vi "VA CoAP - Server - Proccess Message - SET Value TO JSON.vi"(8 "error in (no error)":errorcluster, 9 "New Value":string, 10 "Item name":string[](array[string]), 11 "JSON Value in":refnum<class "JSON Value.lvclass">) -> (0 "error out":errorcluster, 3 "JSON Value out":refnum<class "JSON Value.lvclass">)   [LabVIEW 2020]
uses:
  <vilib>/addons/JSON API/JSON Value/JSON Value.lvclass
  <vilib>/addons/JSON API/JSON Scalar/JSON Scalar.lvclass/JSON Scalar.ctl
  <vilib>/addons/JSON API/JSON Scalar/Quote and Escape JSON string.vi
  <vilib>/addons/JSON API/JSON Scalar/JSON Scalar.lvclass
  c:/Program Files (x86)/National Instruments/LabVIEW 2020/vi.lib/addons/JSON API/JSON Value/JSON Value.lvclass
  <vilib>/addons/JSON API/JSON Value/Set Item by name array.vi
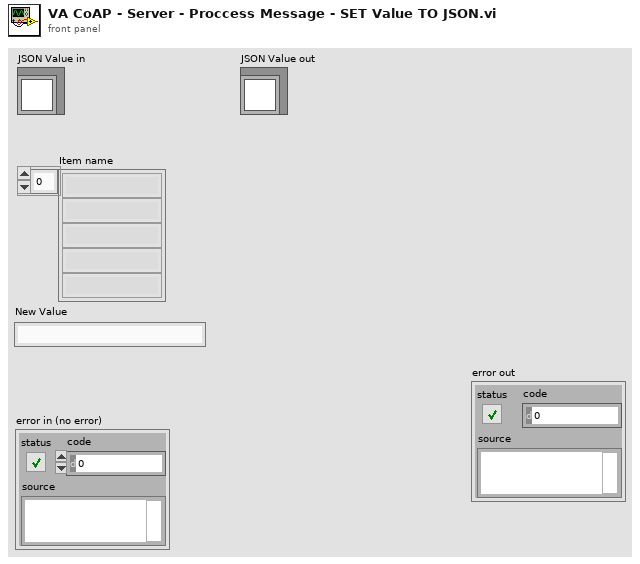
[diagram p1: front panel]
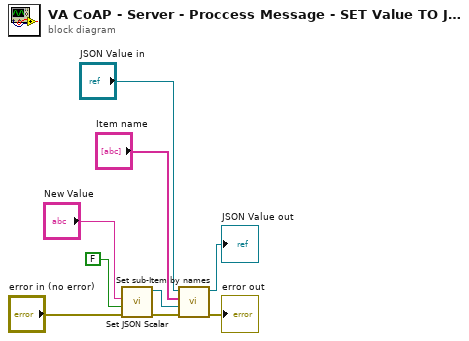
[diagram p0: block diagram]
diagram:
  n1 = call <vilib>:"Set JSON Scalar.vi"("error in (no error)"="error in (no error)", "Set as a JSON string (F)"=FALSE, "LabVIEW Text"="New Value") -> ("error out"=w7:errorcluster, "JSON Scalar out"=w8:refnum<class "JSON Scalar.lvclass">)  [unwired: 7 in]
  n2 = call <vilib>:"Set sub-Item by names.vi"("error in (no error)"=w7, "Value"=w8, "Name Array"="Item name", "JSON Value In"="JSON Value in") -> ("error out"=→"error out":errorcluster, "JSON Value Out"=→"JSON Value out":refnum<class "JSON Value.lvclass">)  [unwired: 5 in, 1 out]
